vi "Continuous Acquisition.vi"() -> ()   [LabVIEW 2019]
uses:
  <vilib>/DAQmx/read.llb/DAQmx Read (Analog Wfm 1Chan NSamp).vi
  <vilib>/DAQmx/create/channels.llb/DAQmx Create Channel (AI-Voltage-Basic).vi
  <vilib>/DAQmx/configure/timing.llb/DAQmx Timing (Sample Clock).vi
  <vilib>/DAQmx/miscellaneous.llb/DAQmx Fill In Error Info.vi
  <resource>/objmgr/daqmx.rc
panel:
  in  "Stop":bool
  out "Actual Sample Rate (Hz)":dbl
  in  "Desired Sample Rate (Hz)":dbl
  in  "Physical Channel":tag
  out "Data":waveform(dbl)(graph)
  in  "Number of Samples":i32
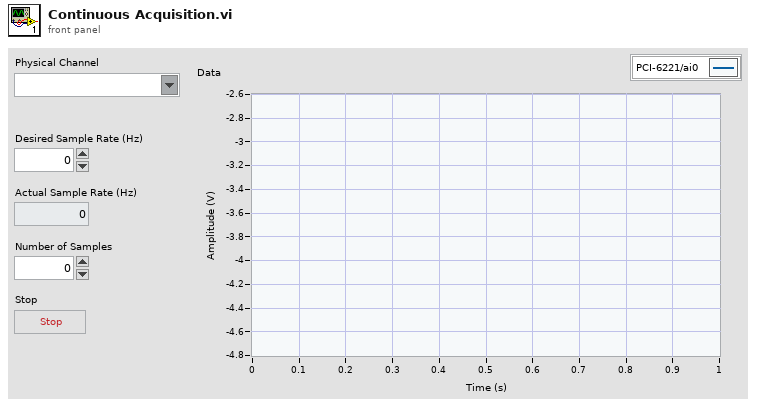
[diagram p1: front panel]
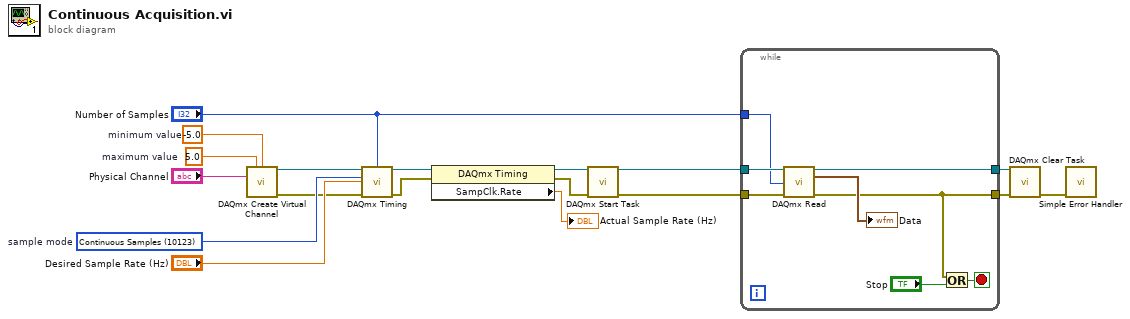
[diagram p0: block diagram]
diagram:
  w1 = -5.0  # minimum value
  w2 = 5.0  # maximum value
  w14 = 10123 items=["Finite Samples"=10178, "Continuous Samples"=10123, "Hardware Timed Single Point"=12522]  # sample mode
  n1 = call-poly <vilib>:"DAQmx Create Virtual Channel.vi"("maximum value"=w2, "minimum value"=w1, "physical channels"="Physical Channel") -> ("task out"=w12:refnum<k21>, "error out"=w11:errorcluster)  [unwired: 11 in]
  n2 = call-poly <vilib>:"DAQmx Timing.vi"("task/channels in"=w12, "sample mode"=w14, "samples per channel"="Number of Samples", "rate"="Desired Sample Rate (Hz)", "error in"=w11) -> ("task out"=w10:refnum<k21>, "error out"=w9:errorcluster)  [unwired: 9 in]
  n3 = property class="DAQmx Timing"(reference=w10, error in=w9) -> (reference out=w8:refnum<k21>, error out=w7:errorcluster, "SampClk.Rate"=→"Actual Sample Rate (Hz)":dbl)
  n4 = call <vilib>:"DAQmx Start Task.vi"("task/channels in"=w8, "error in"=w7) -> ("task out"=w18:refnum<k21>, "error out"=w5:errorcluster)  [unwired: 12 in]
  n5 = while {
    tunnel: "Number of Samples" -> [w22]
    tunnel: w18 -> [w26]
    tunnel: [w25] -> w17
    tunnel: w5 -> [w23]
    tunnel: [w20] -> w16
    stop <- w21 stop-if-true
    n6 = call-poly <vilib>:"DAQmx Read.vi"("task/channels in"=w26, "number of samples per channel"=w22, "error in"=w23) -> ("task out"=w25:refnum<k21>, "data"=→"Data":waveform(dbl), "error out"=w20:errorcluster)  [unwired: 10 in]
    n7 = Or(x=w20, y="Stop") -> (x .or. y?=w21:bool)
  }
  n8 = call <vilib>:"DAQmx Clear Task.vi"("task in"=w17, "error in"=w16) -> ("error out"=w3:errorcluster)  [unwired: 13 in]
  n9 = call <vilib>:"Simple Error Handler.vi"("error in (no error)"=w3) -> ()  [unwired: 4 in, 5 out]
